vi "State Callers.vi"(5 "Calling VI Ref":refnum<vi>, 8 "error in (no error)":errorcluster, 9 "Callers":T1(array[cluster]), 10 "State":string, 11 "JKI SM in":refnum<class "JKI SM.lvclass">) -> (0 "error out":errorcluster)   [LabVIEW 2013]
uses:
  JKI State Machine API/source/JKI SM/JKI SM.lvclass
  JKI State Machine API/source/JKI SM/JKI SM.lvclass/JKI SM.ctl
  <userlib>/_OpenG.lib/error/error.llb/Filter Error Codes (Array)__ogtk.vi
  <vilib>/regexp/Match Regular Expression.xnode
  <userlib>/_OpenG.lib/comparison/comparison.llb/I32 Changed__ogtk.vi
  <userlib>/_OpenG.lib/comparison/comparison.llb/Boolean Changed__ogtk.vi
panel:
  in  "Listbox":i32(listbox)
  in  "OK":bool
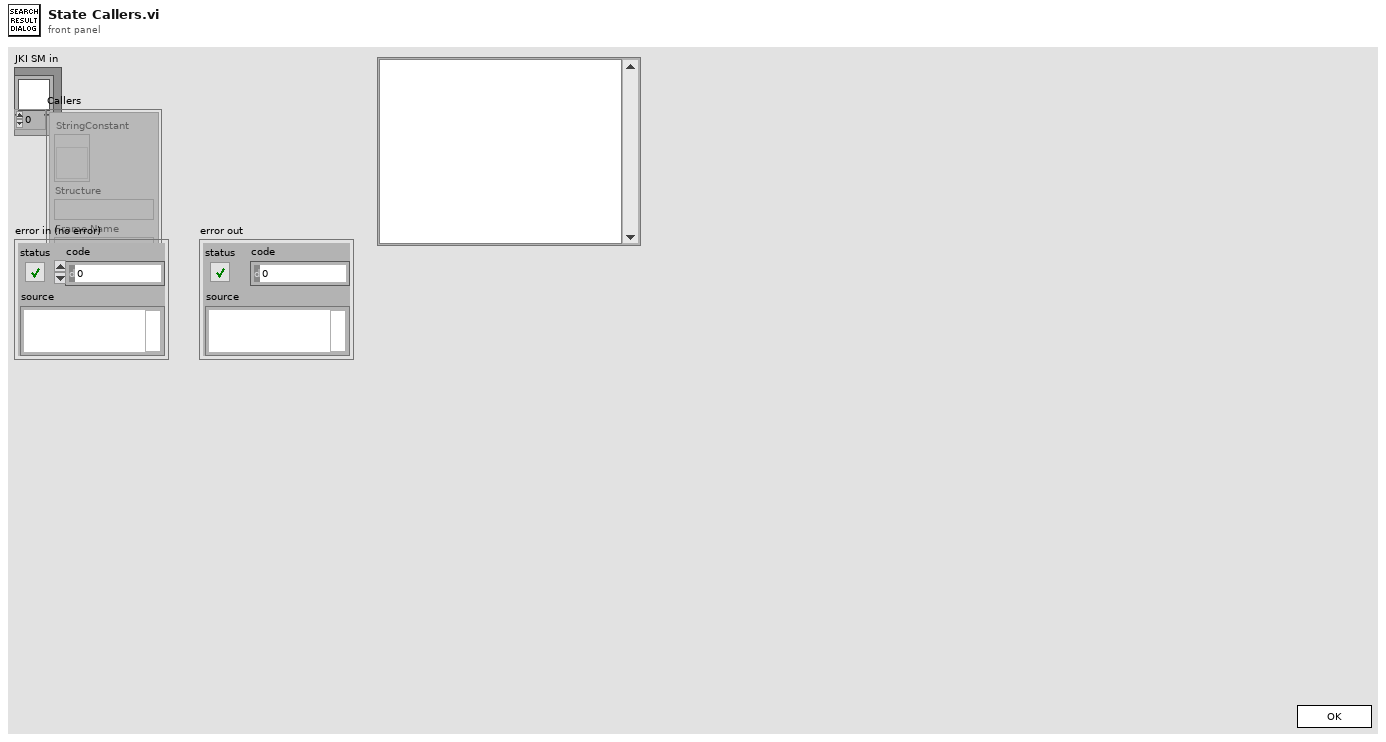
[diagram p1: front panel]
types:
  T1 = cluster{"StringConstant":refnum<vi>, "Structure":string, "Frame Name":string}[]
  T2 = enum32{"Invalid", "Standard", "Closed", "Hidden", "Minimized", "Maximized"}
  T3 = enum32{"invalid app kind", "Development System", "Run Time System", "Student Edition", "Embedded LabVIEW", "Evaluation", "Custom"}
  T4 = enum32{"Invalid", "Default", "Floating", "Floating/Auto-Hide", "Modal"}
  T5 = cluster{"Core":cluster{"Current VI Reference":refnum<vi>, "Close Panel on Exit?":bool}, "Your Boolean data":bool, "Your string data":string, "State":string, "JKI SM out":refnum<class "JKI SM.lvclass">, "Callers":cluster{"StringConstant":refnum<vi>, "Structure":string, "Frame Name":string}[]}
  T6 = cluster{"StringConstant":refnum<vi>, "Structure":string, "Frame Name":string}
  T7 = typedef "LVPoint32TypeDef.ctl" = cluster{"Horizontal":i32, "Vertical":i32}
  T8 = cluster{"Shift":bool, "Ctrl":bool, "Alt":bool, "Cmd":bool, "Opt":bool}
  T9 = cluster{"Current VI Reference":refnum<vi>, "Close Panel on Exit?":bool}
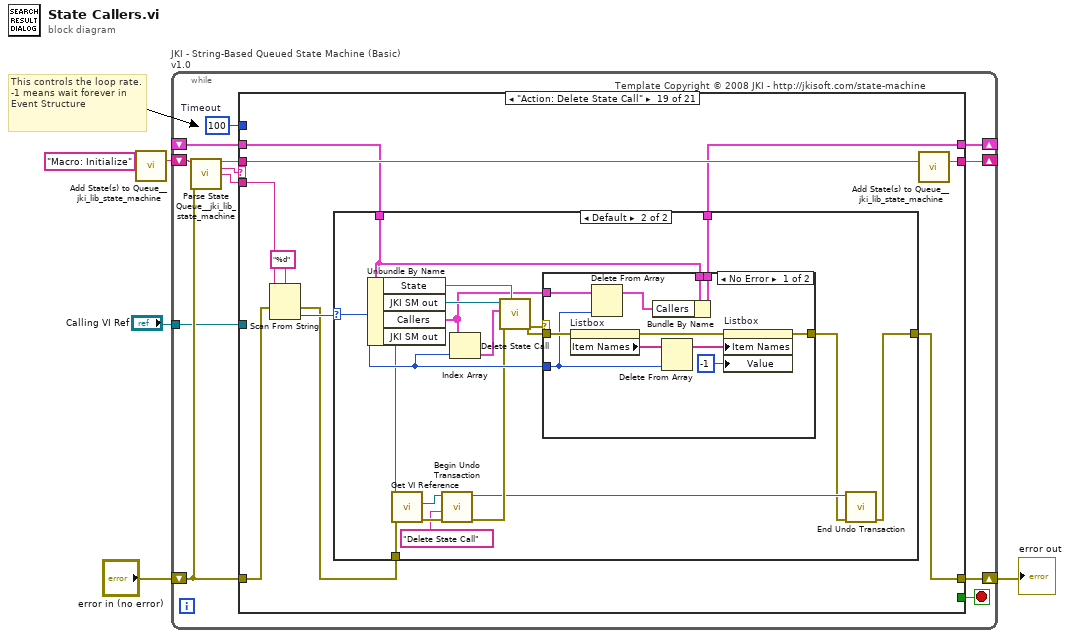
[diagram p0: block diagram]
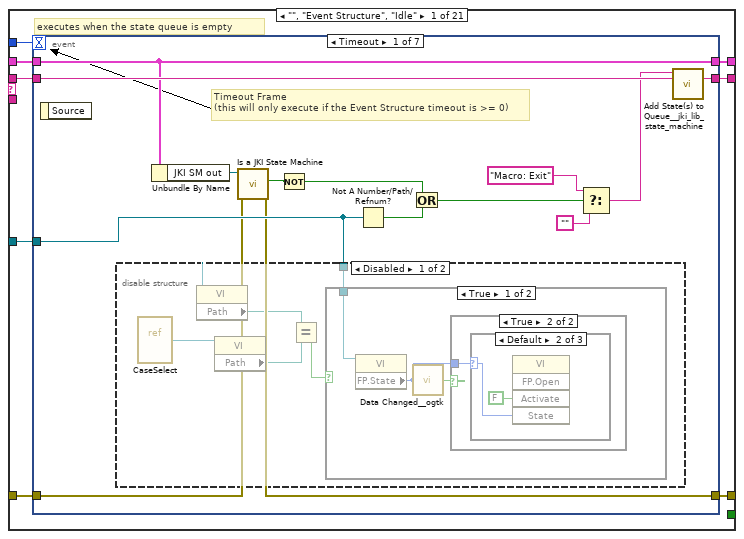
[diagram p2: hidden frame]
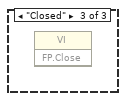
[diagram p5: hidden frame]
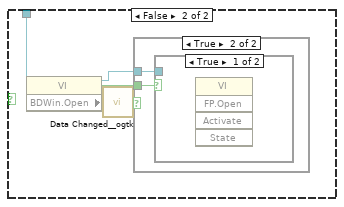
[diagram p6: hidden frame]
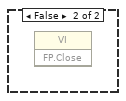
[diagram p8: hidden frame]
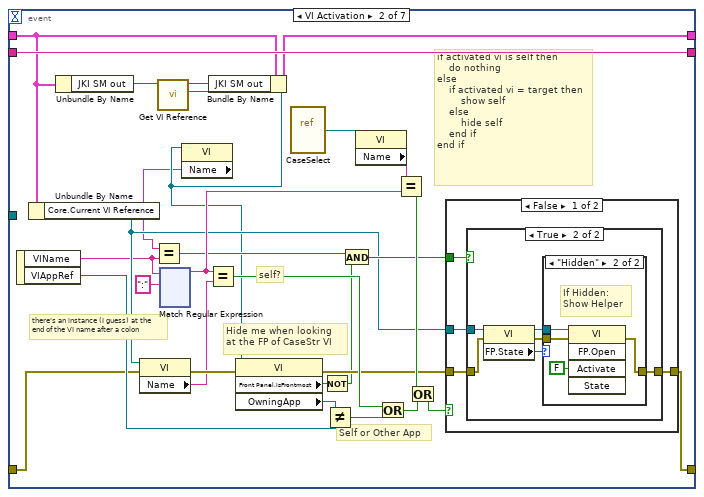
[diagram p10: hidden frame]
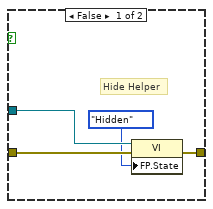
[diagram p11: hidden frame]
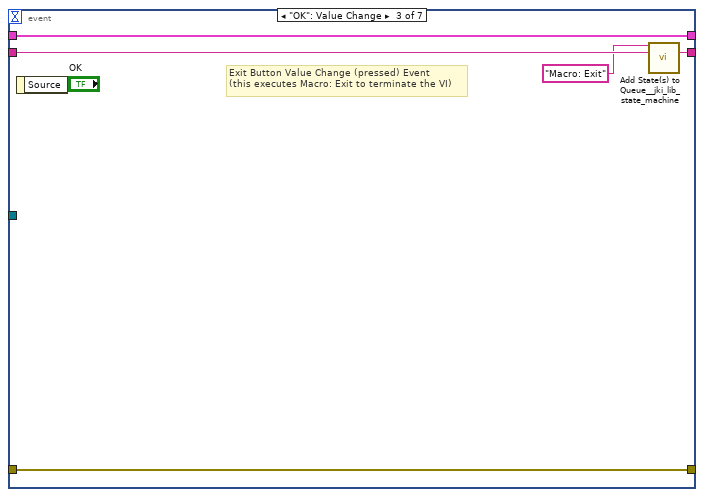
[diagram p14: hidden frame]
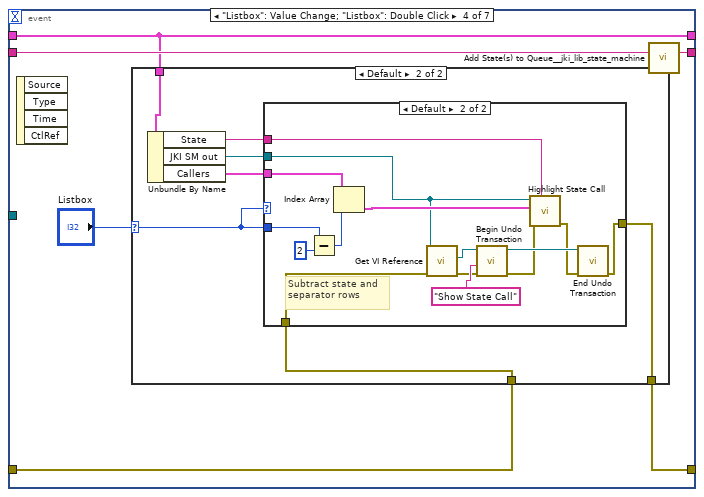
[diagram p15: hidden frame]
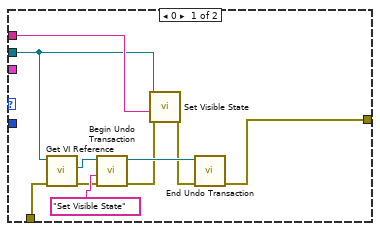
[diagram p17: hidden frame]
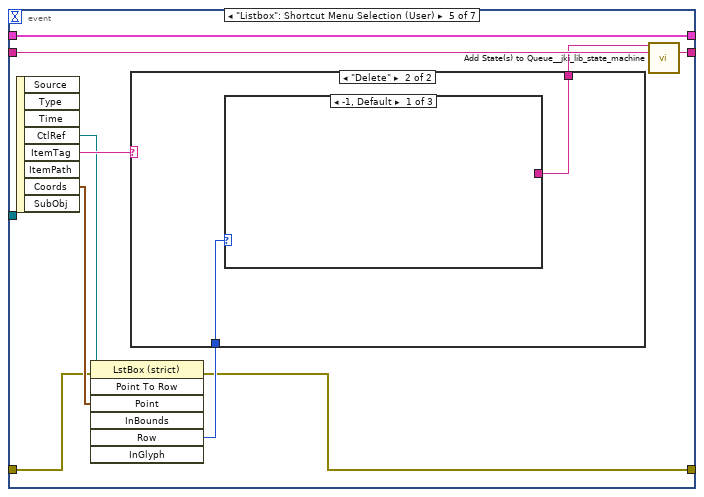
[diagram p18: hidden frame]
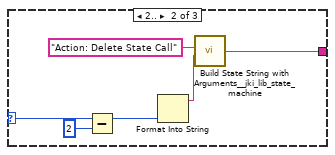
[diagram p20: hidden frame]
diagram:
  # "This controls the loop rate. -1 means wait forever in Event Structure"
  n1 = call <vilib>:"Add State(s) to Queue__jki_lib_state_machine.vi"("State(s) in (\"\")"="Macro: Initialize") -> ("States Out"=w5:string)  [unwired: 14 in]
  n2 = while "JKI - String-Based Queued State Machine (Basic) v1.0" {
    shift-right: [w10] -> _
    shift-left: _ -> [w9]
    shift-right: [w13] -> w3
    shift-left: "error in (no error)" -> [w7]
    shift-right: [w12] -> _
    shift-left: w5 -> [w14]
    tunnel: "Calling VI Ref" -> [w6]
    stop <- w11 stop-if-true
    w8 = 100  # Timeout
    # "Template Copyright © 2008 JKI - http://jkisoft.com/state-machine"
    n3 = call <vilib>:"Parse State Queue__jki_lib_state_machine.vi"("State Queue"=w14, "Error In (no error)"=w7) -> ("Remaining States"=w16:string, "Current State"=w17:string, "Arguments"=w15:string)  [unwired: 11 in]
    n4 = case shown="\"Action: Delete State Call\"" w17 {
      selector: w17 -> [_ _ w369 _ _ _ _ _ _ _ _ _ _ _ _ _ _ _ _ _ _]
      tunnel: w16 -> [w25 w368 w373 w393 w404 w409 w413 w427 w441 w447 w465 w480 w499 w510 w539 w544 w554 w558 w568 w614 w633]
      tunnel: w15 -> [_ _ _ _ _ _ _ _ _ _ _ _ w494 w504 _ _ _ _ w566 _ _]
      tunnel: w9 -> [w23 w365 w371 w385 w401 w407 w410 _ w438 w444 w462 w474 w497 w506 w536 w542 w551 w555 w560 w608 w630]
      tunnel: [w22 w366 w375 w380 errorcluster {"status"=FALSE, "code"=0, "source"=""} ("error out") w406 w411 w417 w434 w445 w463 w471 w495 w507 w537 w540 w552 w556 w561 w611 w631] -> w13
      tunnel: w7 -> [w21 w366 w374 w381 w399 w406 w411 w414 w429 w445 w463 w472 w496 w508 w537 w540 w552 w556 w564 w612 w631]
      tunnel: [w24 w367 w372 w392 w403 w408 w412 w426 w440 w446 w464 w479 w498 w509 w538 w543 w553 w557 w567 w613 w632] -> w12
      tunnel: [_ _ _ _ _ TRUE _ _ _ _ _ _ _ _ _ _ _ _ _ _ _] -> w11
      tunnel: [w20 w365 w371 w391 w401 w407 w410 w425 w438 w444 w462 w474 w497 w506 w536 w542 w551 w555 w559 w610 w630] -> w10
      tunnel: w8 -> [w19 _ _ _ _ _ _ _ _ _ _ _ _ _ _ _ _ _ _ _ _]
      tunnel: w6 -> [w18 _ _ _ _ _ _ _ _ _ _ _ _ _ _ _ _ _ _ _ _]
      frame "", "Event Structure", "Idle" {
        # "executes when the state queue is empty"
        n5 = event shown="[0] Timeout" {
          selector: _ -> [_ _ _ _ _ _ _]
          dyn-events: _ -> [_ _ _ _ _ _ _]
          timeout: w19 -> [_ _ _ _ _ _ _]
          tunnel: w25 -> [w39 w85 w221 w227 w270 w290 w364]
          tunnel: [w38 w85 w220 w226 w269 w289 w363] -> w24
          tunnel: w23 -> [w33 w59 w218 w225 w262 w288 w361]
          tunnel: [w28 w60 w219 w223 w261 w283 w362] -> w22
          tunnel: w21 -> [w29 w61 w219 w224 w264 w284 w362]
          tunnel: [w33 w58 w218 w225 w262 w288 w361] -> w20
          tunnel: w18 -> [w34 _ _ _ _ _ _]
          event Timeout {
            # "Timeout Frame\n(this will only execute if the Event Structure timeout is >= 0)"
            n6 = event-data() -> ()  [unwired: 1 in, 1 out]
            n7 = disable-structure shown="Disabled" {
              disable-tunnel: w34 -> [w40 _]
              frame Disabled {
                n8 = vi-ref "CaseSelect.vi"() -> (w42:refnum<vi>)
                n9 = property class="VI"(reference=w40) -> ("Path"=w41:path)  [unwired: 1 in, 2 out]
                n10 = property class="VI"(reference=w42) -> ("Path"=w44:path)  [unwired: 1 in, 2 out]
                n11 = Equal?(x=w41, y=w44) -> (x = y?=w43:bool)
                n12 = case shown="True" w43 {
                  tunnel: w40 -> [w45 w52]
                  frame True {
                    n13 = property class="VI"(reference=w45) -> ("FP.State"=w46:T2)  [unwired: 1 in, 2 out]
                    n14 = call-poly <userlib>:"Data Changed__ogtk.vi"("I32"=w46) -> ("Changed"=w47:bool)
                    n15 = case shown="True" w47 {
                      tunnel: w46 -> [_ w48]
                      frame False {
                      }
                      frame True {
                        n16 = case shown="Default" w48 {
                          selector: w48 -> [_ w49 _]
                          frame "Invalid" {
                          }
                          frame Default {
                            n17 = invoke class="VI" method="FP.Open"("Activate"=FALSE ("Activate?"), "State"=w49) -> ()  [unwired: 3 in, 5 out]
                          }
                          frame "Closed" {
                            n18 = invoke class="VI" method="FP.Close"() -> ()  [unwired: 3 in, 3 out]
                          }
                        }
                      }
                    }
                  }
                  frame False {
                    n19 = property class="VI"(reference=w52) -> (reference out=w51:refnum<vi>, "BDWin.Open"=w53:bool)  [unwired: 1 in, 1 out]
                    n20 = call-poly <userlib>:"Data Changed__ogtk.vi"("Boolean"=w53) -> ("Changed"=w54:bool)
                    n21 = case shown="True" w54 {
                      tunnel: w53 -> [_ w56]
                      tunnel: w51 -> [_ w55]
                      frame False {
                      }
                      frame True {
                        n22 = case shown="True" w56 {
                          tunnel: w55 -> [_ _]
                          frame True {
                            n23 = invoke class="VI" method="FP.Open"() -> ()  [unwired: 5 in, 5 out]
                          }
                          frame False {
                            n24 = invoke class="VI" method="FP.Close"() -> ()  [unwired: 3 in, 3 out]
                          }
                        }
                      }
                    }
                  }
                }
              }
              frame Enabled {
              }
            }
            n25 = Unbundle By Name(w33) -> ("JKI SM out"=w32:refnum<class "JKI SM.lvclass">)
            n26 = call "Is a JKI State Machine.vi"("error in (no error)"=w29, "JKI SM in"=w32) -> ("error out"=w28:errorcluster, "Is a JKI State Machine"=w31:bool)  [unwired: 7 in, 1 out]
            n27 = Not(x=w31) -> (.not. x?=w30:bool)
            n28 = Not A Number/Path/Refnum?(number/path/refnum=w34) -> (NaN/Path/Refnum?=w27:bool)
            n29 = Or(x=w30, y=w27) -> (x .or. y?=w26:bool)
            n30 = Select(t="Macro: Exit", s=w26, f="") -> (s? t:f=w35:string)
            n31 = call <vilib>:"Add State(s) to Queue__jki_lib_state_machine.vi"("State(s) in Front (\"\")"=w35, "State(s) in (\"\")"=w39) -> ("States Out"=w38:string)  [unwired: 13 in]
          }
          event VI Activation {
            # "Self or Other App"
            # "self?"
            # "Hide me when looking\nat the FP of CaseStr VI"
            # "there's an instance (I guess) at the\nend of the VI name after a colon"
            # "if activated vi is self then\n    do nothing\nelse\n    if activated vi = target then\n        show self\n    else\n        hide self\n    end if\nend if"
            n32 = event-data() -> ("VIName"=w63:string, "VIAppRef"=w62:refnum<vi>)  [unwired: 1 in]
            n33 = Unbundle By Name(w59) -> ("Core.Current VI Reference"=w70:refnum<vi>)
            n34 = Unbundle By Name(w59) -> ("JKI SM out"=w66:refnum<class "JKI SM.lvclass">)
            n35 = property class="VI"(reference=w70, error in=w61) -> (error out=w74:errorcluster, "Name"=w69:string)  [unwired: 1 out]
            n36 = call "Get VI Reference.vi"("JKI SM in"=w66) -> ("VI"=w65:refnum<vi>, "JKI SM out"=w57:refnum<class "JKI SM.lvclass">)  [unwired: 8 in, 1 out]
            n37 = xnode "Match Regular Expression"("input string"=w63, "regular expression"=":") -> ("before match"=w81:string)  [unwired: 3 in, 5 out]
            n38 = property class="VI"(reference=w65) -> ("Name"=w64:string)  [unwired: 1 in, 2 out]
            n39 = Equal?(x=w64, y=w63) -> (x = y?=w67:bool)
            n40 = Equal?(x=w81, y=w69) -> (x = y?=w78:bool)
            n41 = Bundle By Name(cluster=w59, "JKI SM out"=w57) -> (w58:T5)
            n42 = property class="VI"(reference=w65, error in=w74) -> (error out=w73:errorcluster, "Front Panel.IsFrontmost"=w71:bool, "OwningApp"=w76:refnum<vi>)  [unwired: 1 out]
            n43 = vi-ref "CaseSelect.vi"() -> (w79:refnum<vi>)
            n44 = Not(x=w71) -> (.not. x?=w72:bool)
            n45 = Not Equal?(x=w76, y=w62) -> (x != y?=w77:bool)
            n46 = And(x=w67, y=w72) -> (x .and. y?=w75:bool)
            n47 = property class="VI"(reference=w79) -> ("Name"=w80:string)  [unwired: 1 in, 2 out]
            n48 = Or(x=w78, y=w77) -> (x .or. y?=w83:bool)
            n49 = Equal?(x=w80, y=w81) -> (x = y?=w82:bool)
            n50 = Or(x=w82, y=w83) -> (x .or. y?=w84:bool)
            n51 = case shown="False" w84 {
              tunnel: w73 -> [w89 w105]
              tunnel: [w87 w105] -> w60
              tunnel: w70 -> [w88 _]
              tunnel: w75 -> [w86 _]
              frame False {
                n52 = case shown="True" w86 {
                  tunnel: w89 -> [w93 w98]
                  tunnel: w88 -> [w92 w99]
                  tunnel: [w91 w96] -> w87
                  frame False {
                    # "Hide Helper"
                    n53 = property class="VI"(reference=w92, error in=w93, "FP.State"=T2."Hidden" ("Front Panel Window:State")) -> (error out=w91:errorcluster)  [unwired: 1 out]
                  }
                  frame True {
                    n54 = property class="VI"(reference=w99, error in=w98) -> (reference out=w95:refnum<vi>, error out=w94:errorcluster, "FP.State"=w97:T2)
                    n55 = case shown="\"Hidden\"" w97 {
                      tunnel: [w100 w104] -> w96
                      tunnel: w95 -> [_ w103]
                      tunnel: w94 -> [w100 w102]
                      frame Default {
                      }
                      frame "Hidden" {
                        # "If Hidden:\nShow Helper"
                        n56 = invoke class="VI" method="FP.Open"(reference=w103, error in=w102, "Activate"=FALSE ("Activate?")) -> (error out=w104:errorcluster)  [unwired: 2 in, 4 out]
                      }
                    }
                  }
                }
              }
              frame True {
              }
            }
          }
          event "OK": Value Change {
            # "Exit Button Value Change (pressed) Event\n(this executes Macro: Exit to terminate the VI)"
            n57 = event-data() -> ()  [unwired: 1 in, 1 out]
            n58 = call <vilib>:"Add State(s) to Queue__jki_lib_state_machine.vi"("State(s) in Front (\"\")"="Macro: Exit", "State(s) in (\"\")"=w221) -> ("States Out"=w220:string)  [unwired: 13 in]
          }
          event "Listbox": Value Change; "Listbox": Double Click {
            n59 = event-data() -> ()  [unwired: 1 in, 4 out]
            n60 = case shown="Default" "Listbox" {
              selector: "Listbox" -> [_ w229]
              tunnel: w225 -> [_ w235]
              tunnel: w224 -> [w228 w232]
              tunnel: [w228 w231] -> w223
              frame -1 {
              }
              frame Default {
                n61 = Unbundle By Name(w235) -> ("State"=w230:string, "JKI SM out"=w233:refnum<class "JKI SM.lvclass">, "Callers"=w234:T1)
                n62 = case shown="Default" w229 {
                  tunnel: w234 -> [_ w260]
                  tunnel: w233 -> [w239 w251]
                  tunnel: w232 -> [w240 w247]
                  tunnel: w229 -> [_ w256]
                  tunnel: [w236 w248] -> w231
                  tunnel: w230 -> [w245 w258]
                  frame 0 {
                    n63 = call "Get VI Reference.vi"("error in (no error)"=w240, "JKI SM in"=w239) -> ("error out"=w243:errorcluster, "VI"=w242:refnum<vi>)  [unwired: 7 in, 1 out]
                    n64 = call "Begin Undo Transaction.vi"("error in (no error)"=w243, "Action"="Set Visible State", "VI in"=w242) -> ("error out"=w238:errorcluster, "VI out"=w241:refnum<vi>)  [unwired: 7 in]
                    n65 = call "Set Visible State.vi"("error in (no error)"=w238, "State Name"=w245, "JKI SM in"=w239) -> ("error out"=w237:errorcluster)  [unwired: 7 in, 1 out]
                    n66 = call "End Undo Transaction.vi"("error in (no error)"=w237, "VI in"=w241) -> ("error out"=w236:errorcluster)  [unwired: 8 in, 1 out]
                  }
                  frame Default {
                    # "Subtract state and separator rows"
                    n67 = Subtract(x=w256, y=2) -> (x-y=w255:i32)
                    n68 = Index Array(array=w260, index=w255) -> (element=w259:T6)
                    n69 = call "Get VI Reference.vi"("error in (no error)"=w247, "JKI SM in"=w251) -> ("error out"=w253:errorcluster, "VI"=w252:refnum<vi>)  [unwired: 7 in, 1 out]
                    n70 = call "Begin Undo Transaction.vi"("error in (no error)"=w253, "Action"="Show State Call", "VI in"=w252) -> ("error out"=w246:errorcluster, "VI out"=w250:refnum<vi>)  [unwired: 7 in]
                    n71 = call "Highlight State Call.vi"("State"=w258, "error in (no error)"=w246, "Cluster"=w259, "JKI SM in"=w251) -> ("error out"=w249:errorcluster)  [unwired: 6 in, 1 out]
                    n72 = call "End Undo Transaction.vi"("error in (no error)"=w249, "VI in"=w250) -> ("error out"=w248:errorcluster)  [unwired: 8 in, 1 out]
                  }
                }
              }
            }
            n73 = call <vilib>:"Add State(s) to Queue__jki_lib_state_machine.vi"("State(s) in (\"\")"=w227) -> ("States Out"=w226:string)  [unwired: 14 in]
          }
          event "Listbox": Shortcut Menu Selection (User) {
            n74 = event-data() -> ("CtlRef"=w267:refnum<vi>, "ItemTag"=w268:string, "Coords"=w266:T7)  [unwired: 1 in, 5 out]
            n75 = invoke class="LstBox (strict)" method="Point To Row"(reference=w267, error in=w264, "Point"=w266) -> (error out=w261:errorcluster, "Row"=w265:i32)  [unwired: 4 in, 5 out]
            n76 = case shown="\"Delete\"" w268 {
              tunnel: w265 -> [_ w272]
              tunnel: [_ w271] -> w263
              frame Default {
              }
              frame "Delete" {
                n77 = case shown="-1, Default" w272 {
                  selector: w272 -> [_ w275 _]
                  tunnel: [_ w276 w279] -> w271
                  frame -1, Default {
                  }
                  frame 2.. {
                    n78 = Subtract(x=w275, y=2) -> (x-y=w274:i32)
                    n79 = Format Into String(w274) -> (resulting string=w277:string)  [unwired: 3 in, 1 out]
                    n80 = call <vilib>:"Build State String with Arguments__jki_lib_state_machine.vi"("Arguments (\"\")"=w277, "State"="Action: Delete State Call") -> ("State with Arguments"=w276:string)  [unwired: 4 in]
                  }
                  frame 0 {
                    n81 = call <vilib>:"Build State String with Arguments__jki_lib_state_machine.vi"("State"="Action: Delete State") -> ("State with Arguments"=w279:string)  [unwired: 5 in]
                  }
                }
              }
            }
            n82 = call <vilib>:"Add State(s) to Queue__jki_lib_state_machine.vi"("State(s) in Front (\"\")"=w263, "State(s) in (\"\")"=w270) -> ("States Out"=w269:string)  [unwired: 13 in]
          }
          event Key Down? {
            n83 = event-data() -> ("Char"=w287:i16, "ScanCode"=w282:i16, "PlatMods"=w286:T8)  [unwired: 1 in, 7 out]
            n84 = case shown="Default" w282 {
              tunnel: w288 -> [_ w308]
              tunnel: w287 -> [_ w306]
              tunnel: w286 -> [_ w303]
              tunnel: [_ w301] -> w285
              tunnel: w284 -> [w292 w299]
              tunnel: [w292 w298] -> w283
              tunnel: [w291 _] -> w281
              frame 83 {
                n85 = local read "Listbox"() -> (w293:i32)
                n86 = case shown="Default" w293 {
                  selector: w293 -> [_ w294]
                  tunnel: [_ w295] -> w291
                  frame -1 {
                  }
                  frame Default {
                    n87 = Format Into String(w294) -> (resulting string=w296:string)  [unwired: 3 in, 1 out]
                    n88 = call <vilib>:"Build State String with Arguments__jki_lib_state_machine.vi"("Arguments (\"\")"=w296, "State"="Action: Delete State Call") -> ("State with Arguments"=w295:string)  [unwired: 4 in]
                  }
                }
              }
              frame Default {
                n89 = Unbundle By Name(w308) -> ("JKI SM out"=w300:refnum<class "JKI SM.lvclass">, "Callers"=w307:T1)
                n90 = Build Array(w306) -> (w305:i16[])
                n91 = Unbundle By Name(w303) -> ("Ctrl"=w302:bool)
                n92 = Byte Array To String(unsigned byte array=w305) -> (string=w304:string)
                n93 = case shown="True" w302 {
                  tunnel: w307 -> [_ w317]
                  tunnel: w304 -> [_ w316]
                  tunnel: w303 -> [_ w315]
                  tunnel: [_ w314] -> w301
                  tunnel: w300 -> [_ w312]
                  tunnel: [w309 w311] -> w298
                  tunnel: w299 -> [w309 w310]
                  frame False {
                  }
                  frame True {
                    n94 = To Upper Case(1:w316) -> (0:w313:string)
                    n95 = case shown="\"Z\"" w313 {
                      tunnel: w317 -> [_ w332 w342 _]
                      tunnel: w315 -> [_ w327 _ w351]
                      tunnel: [_ TRUE TRUE TRUE] -> w314
                      tunnel: w312 -> [_ _ w335 w348]
                      tunnel: [w318 w325 w333 w345] -> w311
                      tunnel: w310 -> [w318 w325 w334 w349]
                      frame Default {
                      }
                      frame "G" {
                        w320 = 2 ("y")
                        n96 = local read "Listbox"() -> (w322:i32)
                        n97 = Unbundle By Name(w327) -> ("Shift"=w328:bool)
                        n98 = Array Size(array=w332) -> (size(s)=w319:i32)
                        n99 = Subtract(x=w322, y=w320) -> (x-y=w321:i32)
                        n100 = Decrement(x=w321) -> (x-1=w330:i32)
                        n101 = Increment(x=w321) -> (x+1=w331:i32)
                        n102 = Select(t=w330, s=w328, f=w331) -> (s? t:f=w329:i32)
                        n103 = Quotient & Remainder(x=w329, y=w319) -> (x-y*floor(x/y)=w324:i32)  [unwired: 1 out]
                        n104 = Add(x=w324, y=w320) -> (x+y=w323:i32)
                        n105 = property on="Listbox" class="LstBox (strict)"("Val(Sgnl)"=w323) -> ()  [unwired: 2 in, 2 out]
                      }
                      frame "F" {
                        n106 = local read "Listbox"() -> (w343:i32)
                        n107 = Index Array(array=w342, index=w343) -> (element=w341:T6)
                        n108 = Unbundle By Name(w341) -> ("Frame Name"=w337:string)
                        n109 = control-ref of="This VI"() -> (w336:refnum<vi>)
                        n110 = call "Find All Callers of State.vi"("error in (no error)"=w334, "State Name"=w337, "JKI SM in"=w335) -> ("error out"=w338:errorcluster, "Callers"=w339:T1, "JKI SM out"=w340:refnum<class "JKI SM.lvclass">)  [unwired: 6 in]
                        n111 = call "Open Search Results Dialog.vi"("VI Refnum"=w336, "error in (no error)"=w338, "Callers"=w339, "State"=w337, "JKI SM in"=w340) -> ("error out"=w333:errorcluster)  [unwired: 6 in]
                      }
                      frame "Z" {
                        # "Override Ctrl+Z and Ctrl+Shift+Z\n(Handle them here and target the user's VI)"
                        n112 = call "Get VI Reference.vi"("error in (no error)"=w349, "JKI SM in"=w348) -> ("error out"=w346:errorcluster, "VI"=w347:refnum<vi>)  [unwired: 7 in, 1 out]
                        n113 = Unbundle By Name(w351) -> ("Shift"=w350:bool)
                        n114 = case shown="False" w350 {
                          tunnel: w347 -> [w355 w358]
                          tunnel: w346 -> [w353 w357]
                          tunnel: [w354 w356] -> w345
                          frame False {
                            n115 = invoke class="VI" method="Transaction.Undo"(reference=w355, error in=w353) -> (error out=w354:errorcluster)  [unwired: 1 in, 2 out]
                          }
                          frame True {
                            n116 = invoke class="VI" method="Transaction.Redo"(reference=w358, error in=w357) -> (error out=w356:errorcluster)  [unwired: 1 in, 2 out]
                          }
                        }
                      }
                    }
                  }
                }
              }
            }
            n117 = event-data("Discard?"=w285) -> ()  [unwired: 1 in, 1 out]
            n118 = call <vilib>:"Add State(s) to Queue__jki_lib_state_machine.vi"("State(s) in Front (\"\")"=w281, "State(s) in (\"\")"=w290) -> ("States Out"=w289:string)  [unwired: 13 in]
          }
          event Panel Close? {
            # "Discard the event because we'll close the front panel ourselves in Macro: Exit"
            # "Close Panel button (pressed) Event\n(this executes Macro: Exit to terminate the VI)"
            n119 = event-data() -> ()  [unwired: 1 in, 1 out]
            n120 = event-data("Discard?"=TRUE) -> ()  [unwired: 1 in, 1 out]
            n121 = call <vilib>:"Add State(s) to Queue__jki_lib_state_machine.vi"("State(s) in Front (\"\")"="Macro: Exit", "State(s) in (\"\")"=w364) -> ("States Out"=w363:string)  [unwired: 13 in]
          }
        }
      }
      frame "---------- Core ----------" {
        # "Do not put any code in this frame.\n(it is a separator no-op)"
        n122 = call <vilib>:"Add State(s) to Queue__jki_lib_state_machine.vi"("State(s) in (\"\")"=w368) -> ("States Out"=w367:string)  [unwired: 14 in]
      }
      frame Default {
        w378 = 42 items=["No error", "Argument error", "Memory is full", "Out of zone", "End of file", "File already open", "Generic file I/O error", "File not found", "File permission error", "Disk is full", "Duplicate path", "Too many files open", "System feature not enabled", "Resource file not found", "Cannot add resource", "Resource not found", "Image not found", "Image memory error", "Pen does not exist", "Config type invalid", "Config token not found", "Config parse error", "Config memory error", "Bad external code format", "Bad external code offset", "External code not present", "Null window", "Destroy window error", "Null menu", "Print aborted", "Bad print record", "Print driver error", "Windows error during printing", "Memory error during printing", "Print dialog error", "Generic print error", "Invalid device refnum", "Device not found", "Device parameter error", "Device unit error", "Cannot open device", "Device call aborted", "Generic error", "Cancelled by user", "Object ID too low", "Object ID too high", "Object not in heap", "Unknown heap", "Unknown object (invalid DefProc)", "Unknown object (DefProc not in table)", "Message out of range", "Invalid (null) method", "Unknown message", "Manager call not supported", "Bad address", "Network operation in progress", "Network operation timed out", "Connection is busy", "Network attribute not supported", "Network error", "Address in use", "System out of memory", "Connection aborted", "Connection refused", "Not connected", "Already connected", "Connection closed", "Initialization error (interapplication manager)", "Bad occurrence", "Wait on unbound occurrence handler", "Occurrence queue overflow", "Datalog type conflict", "Unused", "Unrecognized type (interapplication manager)", "Memory corrupt", "Failed to make temporary DLL", "Old CIN version", "Drag socket not found", "Failed to load drop-object", "Failed to register OLE object", "Failed to release OLE object", "Format specifier type mismatch", "Unknown format specifier", "Too few format specifiers", "Too many format specifiers", "Scan failed", "Newer CIN version", "Error converting to variant", "Runtime menu error", "Password tampered", "Variant attribute not found", "Incompatible variant data type", "Event data is not available", "Event Store is not present", "Occurrence is not found", "Event Queue is not created", "Event info is not available", "Refnum passed is NULL", "Error retrieving Class GUID", "Error retrieving CoClass GUID", "Error retrieving TypeLib GUID.", "Bad built application magic bytes.", "Specific driver is different from the specific driver associated with the Logical Name.", "There is no session opened to the class driver.", "Max Error", "MAX - Error with config objects", "MAX - Error loading configuration", "MAX - Group not supported"]
        # "Current State"
        # "Do not delete, rename, or modify this frame.\n(this is used to capture unhandled states and typos)"
        # "Handle mistyped state name (developer tool)"
        n123 = Format Into String(format string="Software Exception: Unhandled State \"%s\"." ("message"), error in=w374, w369) -> (resulting string=w377:string, error out=w376:errorcluster)  [unwired: 1 in]
        n124 = call <vilib>:"Error Cluster From Error Code.vi"("show call chain? (False)"=TRUE, "error in (no error)"=w376, "error message (\"\")"=w377, "error code (0)"=w378) -> ("error out"=w375:errorcluster)  [unwired: 5 in]
        n125 = call <vilib>:"Add State(s) to Queue__jki_lib_state_machine.vi"("State(s) in (\"\")"=w373) -> ("States Out"=w372:string)  [unwired: 14 in]
      }
      frame "Initialize Core Data" {
        # "Do not delete, rename, or modify this frame.\n(this is used to determine panel behavior on exit)"
        # "originally closed?"
        # "exe?"
        # "If panel starts closed or is an EXE, then close it when we exit"
        n126 = property class="VI"() -> ("Clone Name"=w383:string)  [unwired: 2 in, 2 out]
        n127 = Open VI Reference(vi path=w383, error in (no error)=w381) -> (vi reference=w382:refnum<vi>, error out=w380:errorcluster)  [unwired: 4 in]
        n128 = property class="VI"() -> ("Front Panel.Open"=w390:bool)  [unwired: 2 in, 2 out]
        n129 = property class="App"() -> ("App.Kind"=w389:T3)  [unwired: 2 in, 2 out]
        n130 = Not(x=w390) -> (.not. x?=w387:bool)
        n131 = Equal?(x=w389, y=T3."Run Time System" ("Application:Kind")) -> (x = y?=w386:bool)
        n132 = Or(x=w387, y=w386) -> (x .or. y?=w384:bool)
        n133 = Bundle By Name(cluster=w385, "Core.Current VI Reference"=w382, "Core.Close Panel on Exit?"=w384) -> (w391:T5)
        n134 = call <vilib>:"Add State(s) to Queue__jki_lib_state_machine.vi"("State(s) in (\"\")"=w393) -> ("States Out"=w392:string)  [unwired: 14 in]
      }
      frame "Error Handler" {
        w400 = i32[] [1026]  # JKI SM VI Invalid Ref
        # "Unhandled Error -- Display it"
        # "Handle any errors here.\nYou can also output any states to clean-up after errors occur"
        # "Clear error"
        n135 = call-poly <userlib>:"Filter Error Codes__ogtk.vi"("Error In"=w399, "Error Codes to Filter"=w400) -> ("Error Out"=w398:errorcluster, "Error Filtered?"=w397:bool)  [unwired: 7 in, 1 out]
        n136 = call <vilib>:"General Error Handler.vi"("error in (no error)"=w398) -> ()  [unwired: 10 in, 5 out]
        n137 = Select(t="Macro: Exit", s=w397, f="") -> (s? t:f=w394:string)
        n138 = call <vilib>:"Add State(s) to Queue__jki_lib_state_machine.vi"("State(s) in Front (\"\")"=w394, "State(s) in (\"\")"=w404) -> ("States Out"=w403:string)  [unwired: 13 in]
      }
      frame "Exit" {
        # "Do not put any code in this frame.\n(No errors that occur here will be handled.)"
        n139 = call <vilib>:"Add State(s) to Queue__jki_lib_state_machine.vi"("State(s) in (\"\")"=w409) -> ("States Out"=w408:string)  [unwired: 14 in]
      }
      frame "---------- Data ----------" {
        # "Do not put any code in this frame.\n(It is a separator no-op. You can make a copy of this frame to create a new Data frame)"
        n140 = call <vilib>:"Add State(s) to Queue__jki_lib_state_machine.vi"("State(s) in (\"\")"=w413) -> ("States Out"=w412:string)  [unwired: 14 in]
      }
      frame "Data: Initialize" {
        w422 = T9 {"Current VI Reference"=refnum, "Close Panel on Exit?"=FALSE}  # Core
        w424 = TRUE  # Your Boolean data
        w423 = ""  # Your string data
        # "Open New Ref"
        # "do not delete - used by framework"
        # "Expand Bundle to add new data elements to shift register data."
        # "Add new data here."
        # "Data names and types of shift register data are defined by this bundle."
        # "Initialize the shift-register data, here.\n(data names are defined by what you wire into the bundle function)"
        n141 = call "Get VI Case Structure Reference.vi"("error in (no error)"=w414, "JKI SM in"="JKI SM in") -> ("error out"=w418:errorcluster, "Case Structure ref"=w419:refnum<vi>)  [unwired: 7 in, 1 out]
        n142 = call "Create (From Structure).vi"("error in (no error)"=w418, "Structure"=w419) -> ("error out"=w417:errorcluster, "JKI SM out"=w415:refnum<class "JKI SM.lvclass">)  [unwired: 8 in]
        n143 = Bundle("Core"=w422, "Your Boolean data"=w424, "Your string data"=w423, "State"="State", "JKI SM out"=w415, "Callers"="Callers") -> (w425:T5)  [unwired: 1 in]
        n144 = call <vilib>:"Add State(s) to Queue__jki_lib_state_machine.vi"("State(s) in (\"\")"=w427) -> ("States Out"=w426:string)  [unwired: 14 in]
      }
      frame "Data: Cleanup" {
        # "Ignore Errors\n(e.g. reference already invalid)"
        # "Cleanup any data and references, here.\n(this is called automatically, by the Macro: Exit)"
        n145 = Unbundle By Name(w438) -> ("Core.Current VI Reference"=w439:refnum<vi>, "Callers"=w437:T1, "JKI SM out"=w431:refnum<class "JKI SM.lvclass">)
        n146 = for {
          tunnel: w437 -> [w443] mode=indexing
          tunnel: [w442] -> w436 mode=indexing
          n147 = Unbundle By Name(w443) -> ("StringConstant"=w442:refnum<vi>)
        }
        n148 = Close Reference(reference=w439, error in (no error)=w429) -> (error out=w435:errorcluster)
        n149 = Close Reference(reference=w436, error in (no error)=w429) -> (error out=w433:errorcluster)
        n150 = call "Destroy.vi"("error in (no error)"=w429, "JKI SM in"=w431) -> ("error out"=w430:errorcluster)  [unwired: 9 in]
        n151 = call <userlib>:"Clear All Errors__ogtk.vi"("Upsteam Error (optional)"=w429, "Error In"=w430) -> ("Error Out"=w428:errorcluster)  [unwired: 2 in]
        n152 = call <userlib>:"Clear All Errors__ogtk.vi"("Upsteam Error (optional)"=w429, "Error In"=w433) -> ("Error Out"=w432:errorcluster)  [unwired: 2 in]
        n153 = Merge Errors(w435, w432, w428) -> (w434:errorcluster)
        n154 = call <vilib>:"Add State(s) to Queue__jki_lib_state_machine.vi"("State(s) in (\"\")"=w441) -> ("States Out"=w440:string)  [unwired: 14 in]
      }
      frame "---------- UI ----------" {
        # "Do not put any code in this frame.\n(It is a separator no-op. You can make a copy of this frame to create a new UI frame)"
        n155 = call <vilib>:"Add State(s) to Queue__jki_lib_state_machine.vi"("State(s) in (\"\")"=w447) -> ("States Out"=w446:string)  [unwired: 14 in]
      }
      frame "UI: Initialize" {
        # "Initialize the User Interface, here.\n(this is called automatically, by the Macro: Init)"
        n156 = Unbundle By Name(w462) -> ("Core.Current VI Reference"=w460:refnum<vi>, "State"=w455:string, "Callers"=w461:T1)
        n157 = for {
          tunnel: w461 -> [w470] mode=indexing
          tunnel: [w467] -> w453 mode=indexing
          n158 = Unbundle By Name(w470) -> ("Structure"=w469:string, "Frame Name"=w468:string)
          n159 = Format Into String(format string="%s: %s", w469, w468) -> (resulting string=w467:string)  [unwired: 2 in, 1 out]
        }
        n160 = Format Into String(format string="Find Callers (%s)", w455) -> (resulting string=w458:string)  [unwired: 2 in, 1 out]
        n161 = property class="VI"(reference=w460, "Front Panel.Title"=w458) -> ()  [unwired: 1 in, 2 out]
        n162 = Build Array (concatenate)(w455, "" ("format string"), w453) -> (w454:string[])
        n163 = property on="Listbox" class="LstBox (strict)"("Item Names"=w454, "Value"=-1 ("Listbox")) -> (error out=w452:errorcluster, "Item Symbols"=w451:i32[])  [unwired: 2 in, 1 out]
        n164 = Replace Array Subset(array=w451, new element=-1 ("new element/subarray"), index=1) -> (w450:i32[])
        n165 = property on="Listbox" class="LstBox (strict)"(error in=w452, "Item Symbols"=w450) -> ()  [unwired: 1 in, 2 out]
        n166 = call <vilib>:"Add State(s) to Queue__jki_lib_state_machine.vi"("State(s) in (\"\")"=w465) -> ("States Out"=w464:string)  [unwired: 14 in]
      }
      frame "UI: Pre-Test for 0 or 1 Items" {
        n167 = Unbundle By Name(w474) -> ("JKI SM out"=w475:refnum<class "JKI SM.lvclass">, "State"=w477:string, "Callers"=w476:T1)
        n168 = Array Size(array=w476) -> (size(s)=w478:i32)
        n169 = case shown="1" w478 {
          tunnel: w477 -> [_ w486 w487]
          tunnel: [_ "Macro: Exit" "Macro: Exit"] -> w473
          tunnel: w476 -> [_ _ w492]
          tunnel: w475 -> [_ _ w491]
          tunnel: w472 -> [w481 w482 w489]
          tunnel: [w481 w482 w488] -> w471
          frame Default {
          }
          frame 0 {
            n170 = Format Into String(format string="State %s has no callers.", w486) -> (resulting string=w484:string)  [unwired: 2 in, 1 out]
            n171 = One Button Dialog(message=w484) -> ()  [unwired: 1 in, 1 out]
          }
          frame 1 {
            n172 = Index Array(array=w492) -> (element=w490:T6)  [unwired: 1 in]
            n173 = call "Highlight State Call.vi"("State"=w487, "error in (no error)"=w489, "Cluster"=w490, "JKI SM in"=w491) -> ("error out"=w488:errorcluster)  [unwired: 6 in, 1 out]
          }
        }
        n174 = call <vilib>:"Add State(s) to Queue__jki_lib_state_machine.vi"("State(s) in Front (\"\")"=w473, "State(s) in (\"\")"=w480) -> ("States Out"=w479:string)  [unwired: 13 in]
      }
      frame "UI: Cursor Set" {
        # "Argument"
        # "Set and Unset Cursor Busy.\n(Usage: \"UI: Cursor Set >> Busy|Idle\")"
        n175 = case shown="\"Idle\", Default" w494 {
          tunnel: w496 -> [w501 w503]
          tunnel: [w500 w502] -> w495
          frame "Idle", Default {
            n176 = call <vilib>:"Unset Busy.vi"("error in (no error)"=w501) -> ("error out"=w500:errorcluster)  [unwired: 10 in]
          }
          frame "Busy" {
            n177 = call <vilib>:"Set Busy.vi"("error in (no error)"=w503) -> ("error out"=w502:errorcluster)  [unwired: 9 in, 1 out]
          }
        }
        n178 = call <vilib>:"Add State(s) to Queue__jki_lib_state_machine.vi"("State(s) in (\"\")"=w499) -> ("States Out"=w498:string)  [unwired: 14 in]
      }
      frame "UI: Front Panel State" {
        # "Argument"
        # "Set Front Panel Open or Closed\n(Usage: \"UI: Front Panel State >> Open|Close\")"
        n179 = Unbundle By Name(w506) -> ("Core.Current VI Reference"=w505:refnum<vi>)
        n180 = case shown="\"Open\", Default" w504 {
          tunnel: w508 -> [w514 w530]
          tunnel: [w516 w531] -> w507
          tunnel: w505 -> [w515 w528]
          frame "Open", Default {
            n181 = property class="VI"(reference=w515, error in=w514) -> (reference out=w512:refnum<vi>, error out=w513:errorcluster, "Front Panel.Open"=w511:bool)
            n182 = case shown="False" w511 {
              tunnel: [w519 w525] -> w516
              tunnel: w513 -> [w522 w525]
              tunnel: w512 -> [w521 _]
              frame False {
                # "Setting Floatin here, instead of VI Properties allows the VI to accept keyboard input immediately after openning. (setting it in VI Properties was causing a bug where it wouldn't receive keyboard input until clicking on the VI)"
                n183 = invoke class="VI" method="FP.Open"(reference=w521, error in=w522, "Activate"=TRUE, "State"=T2."Standard") -> (reference out=w518:refnum<vi>, error out=w520:errorcluster)  [unwired: 1 in, 3 out]
                n184 = property class="VI"(reference=w518, error in=w520, "FP.Behavior"=T4."Floating" ("Front Panel Window:Behavior")) -> (error out=w519:errorcluster)  [unwired: 1 out]
              }
              frame True {
              }
            }
          }
          frame "Close" {
            n185 = property class="VI"(reference=w528, error in=w530) -> (reference out=w527:refnum<vi>, error out=w529:errorcluster, "Front Panel.Open"=w526:bool)
            n186 = case shown="True" w526 {
              tunnel: [w532 w535] -> w531
              tunnel: w529 -> [w532 w534]
              tunnel: w527 -> [_ w533]
              frame False {
              }
              frame True {
                n187 = invoke class="VI" method="FP.Close"(reference=w533, error in=w534) -> (error out=w535:errorcluster)  [unwired: 1 in, 2 out]
              }
            }
          }
        }
        n188 = call <vilib>:"Add State(s) to Queue__jki_lib_state_machine.vi"("State(s) in (\"\")"=w510) -> ("States Out"=w509:string)  [unwired: 14 in]
      }
      frame "---------- Macro ----------" {
        # "Do not put any code in this frame.\n(It is a separator no-op. You can make a copy of this frame to create a new Macro frame)"
        n189 = call <vilib>:"Add State(s) to Queue__jki_lib_state_machine.vi"("State(s) in (\"\")"=w539) -> ("States Out"=w538:string)  [unwired: 14 in]
      }
      frame "Macro: Initialize" {
        w541 = "Data: Initialize\nInitialize Core Data\nUI: Pre-Test for 0 or 1 Items\nUI: Initialize\nUI: Front Panel State >> Open"  # Data: Initialize Initialize Core Data UI: Pre-Test for 0 or 1 Items UI: Initialize UI: Front Panel State >> Open
        # "Initialization Macro\n(This is called once, when the VI starts)"
        n190 = call <vilib>:"Add State(s) to Queue__jki_lib_state_machine.vi"("State(s) in Front (\"\")"=w541, "State(s) in (\"\")"=w544) -> ("States Out"=w543:string)  [unwired: 13 in]
      }
      frame "Macro: Exit" {
        # "Exit Macro\n(This is called once, when the VI exits)"
        n191 = Unbundle By Name(w551) -> ("Core.Close Panel on Exit?"=w550:bool)
        n192 = Select(t="UI: Front Panel State >> Close", s=w550, f="") -> (s? t:f=w547:string)
        n193 = call <vilib>:"Add State(s) to Queue__jki_lib_state_machine.vi"("State(s) in (\"\")"=w547, "State(s) at Back (\"\")"="Data: Cleanup\nExit") -> ("States Out"=w545:string)  [unwired: 13 in]
        n194 = call <vilib>:"Add State(s) to Queue__jki_lib_state_machine.vi"("State(s) in Front (\"\")"=w545, "State(s) in (\"\")"=w554) -> ("States Out"=w553:string)  [unwired: 13 in]
      }
      frame "---------- Action ----------" {
        # "Template Separator\n(You can make a copy of, or modify, this frame)"
        n195 = call <vilib>:"Add State(s) to Queue__jki_lib_state_machine.vi"("State(s) in (\"\")"=w558) -> ("States Out"=w557:string)  [unwired: 14 in]
      }
      frame "Action: Delete State Call" {
        n196 = Scan From String(format string="%d", input string=w566, error in=w564) -> (error out=w562:errorcluster, output 1=w563:i32)  [unwired: 2 in, 2 out]
        n197 = case shown="Default" w563 {
          selector: w563 -> [_ w581]
          tunnel: w560 -> [w569 w585]
          tunnel: w562 -> [w570 w576]
          tunnel: [w569 w584] -> w559
          tunnel: [w570 w572] -> w561
          frame -1 {
          }
          frame Default {
            n198 = Unbundle By Name(w585) -> ("State"=w587:string, "JKI SM out"=w586:refnum<class "JKI SM.lvclass">, "Callers"=w582:T1, "JKI SM out"=w578:refnum<class "JKI SM.lvclass">)
            n199 = call "Get VI Reference.vi"("error in (no error)"=w576, "JKI SM in"=w578) -> ("error out"=w575:errorcluster, "VI"=w577:refnum<vi>)  [unwired: 7 in, 1 out]
            n200 = call "Begin Undo Transaction.vi"("error in (no error)"=w575, "Action"="Delete State Call", "VI in"=w577) -> ("error out"=w579:errorcluster, "VI out"=w573:refnum<vi>)  [unwired: 7 in]
            n201 = Index Array(array=w582, index=w581) -> (element=w580:T6)
            n202 = call "Delete State Call.vi"("State"=w587, "error in (no error)"=w579, "Cluster"=w580, "JKI SM in"=w586) -> ("error out"=w583:errorcluster)  [unwired: 6 in, 1 out]
            n203 = case shown="No Error" w583 {
              tunnel: w583 -> [w598 w599]
              tunnel: w581 -> [w590 _]
              tunnel: w585 -> [w594 w600]
              tunnel: [w593 w600] -> w584
              tunnel: w582 -> [w592 _]
              tunnel: [w588 w599] -> w571
              frame No Error {
                n204 = property on="Listbox" class="LstBox (strict)"(error in=w598) -> (error out=w597:errorcluster, "Item Names"=w596:string[])  [unwired: 1 in, 1 out]
                n205 = Delete From Array(array=w592, index=w590) -> (array with subset deleted=w591:T1)  [unwired: 1 in, 1 out]
                n206 = Bundle By Name(cluster=w594, "Callers"=w591) -> (w593:T5)
                n207 = Delete From Array(array=w596, index=w590) -> (array with subset deleted=w595:string[])  [unwired: 1 in, 1 out]
                n208 = property on="Listbox" class="LstBox (strict)"(error in=w597, "Item Names"=w595, "Value"=-1 ("Listbox")) -> (error out=w588:errorcluster)  [unwired: 1 in, 1 out]
              }
              frame Error {
              }
            }
            n209 = call "End Undo Transaction.vi"("error in (no error)"=w571, "VI in"=w573) -> ("error out"=w572:errorcluster)  [unwired: 8 in, 1 out]
          }
        }
        n210 = call <vilib>:"Add State(s) to Queue__jki_lib_state_machine.vi"("State(s) in (\"\")"=w568) -> ("States Out"=w567:string)  [unwired: 14 in]
      }
      frame "Action: Delete State" {
        n211 = Unbundle By Name(w608) -> ("State"=w606:string, "Callers"=w607:T1)
        n212 = Array Size(array=w607) -> (size(s)=w605:i32)
        n213 = Format Into String(format string="Are you sure you want to delete \"%s\" and all %d callers?" ("message"), w606, w605) -> (resulting string=w603:string)  [unwired: 2 in, 1 out]
        n214 = Two Button Dialog(message=w603, 2:"Yes: Delete All" ("T button name (\"OK\")")) -> (T button?=w609:bool)  [unwired: 1 in]
        n215 = case shown="True" w609 {
          tunnel: w608 -> [w615 w629]
          tunnel: w612 -> [w616 w622]
          tunnel: [w615 w629] -> w610
          tunnel: [w616 w619] -> w611
          tunnel: [_ "Macro: Exit"] -> w602
          frame False {
          }
          frame True {
            n216 = Unbundle By Name(w629) -> ("State"=w627:string, "JKI SM out"=w623:refnum<class "JKI SM.lvclass">)
            n217 = call "Get VI Reference.vi"("error in (no error)"=w622, "JKI SM in"=w623) -> ("error out"=w624:errorcluster, "VI"=w617:refnum<vi>)  [unwired: 7 in, 1 out]
            n218 = call "Begin Undo Transaction.vi"("error in (no error)"=w624, "Action"="Delete State", "VI in"=w617) -> ("error out"=w621:errorcluster, "VI out"=w618:refnum<vi>)  [unwired: 7 in]
            n219 = call "Delete State.vi"("Delete Callers? (F: Only Delete Case Structure Frame)"=TRUE, "error in (no error)"=w621, "State Name"=w627, "JKI SM in"=w623) -> ("error out"=w620:errorcluster)  [unwired: 6 in, 1 out]
            n220 = call "End Undo Transaction.vi"("error in (no error)"=w620, "VI in"=w618) -> ("error out"=w619:errorcluster)  [unwired: 8 in, 1 out]
          }
        }
        n221 = call <vilib>:"Add State(s) to Queue__jki_lib_state_machine.vi"("State(s) in Front (\"\")"=w602, "State(s) in (\"\")"=w614) -> ("States Out"=w613:string)  [unwired: 13 in]
      }
      frame "New Category: 2" {
        # "Your code here.\n(You can make a copy of, or modify, this frame)"
        n222 = call <vilib>:"Add State(s) to Queue__jki_lib_state_machine.vi"("State(s) in (\"\")"=w633) -> ("States Out"=w632:string)  [unwired: 14 in]
      }
    }
  }
  "error out" <- w3
